vi "Close Serial Port.vi"(11 "error in (no error)":errorcluster) -> (15 "error out":errorcluster)   [LabVIEW 2024, in "GRBL 1.1.lvlib"]
doc: "This VI close the serial port of the selected controller."
uses:
  GRBL 1.1.lvlib
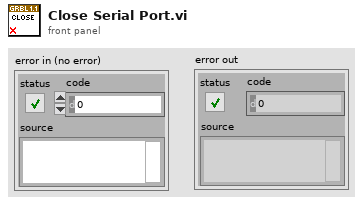
[diagram p1: front panel]
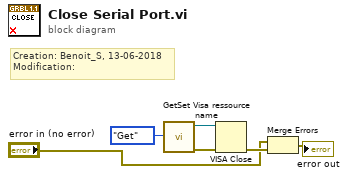
[diagram p0: block diagram]
diagram:
  # "Creation: Benoit_S, 13-06-2018\nModification:"
  n1 = call "GetSet Visa ressource name.vi"("Get/Set"=enum16{"Get", "Set"}."Get") -> ("VISA resource name out"=w2:refnum<visa-resource-name>, "error out"=w3:errorcluster)  [unwired: 13 in]
  n2 = VISA Close(VISA resource name=w2, error in (no error)=w3) -> (error out=w6:errorcluster)
  n3 = Merge Errors("error in (no error)", w6) -> (→"error out":errorcluster)
